vi "SetWindowFullscreen.vi"(8 "No Error":errorcluster, 10 "Fullscreen":bool, 11 "Window [SDL_Window *]":i64 format="%.0x") -> (0 "Error Out":errorcluster)   [LabVIEW 2026, in "SDL3.lvlib" / "Video.lvlib"]
doc: "<B>Summary</B>\nRequest that the window's fullscreen state be changed.\n\n<B>Remarks</B>\nBy default a window in fullscreen state uses borderless fullscreen desktop mode, but a specific exclusive display mode can be set using <B>SDL_SetWindowFullscreenMode()</B>.\n\nOn some windowing systems this request is asynchronous and the new fullscreen state may not have have been applied immediately upon the return of this function. If an immediate change is required, call <B>SDL_SyncWindow()</B> to block until the changes have taken effect.\n\nWhen the window state changes, an <B>SDL_EVENT_WINDOW_ENTER_FULLSCREEN</B> or <B>SDL_EVENT_WINDOW_LEAVE_FULLSCREEN</B> event will be emitted. Note that, as this is just a request, it can be denied by the windowing system."
uses:
  Video.lvlib
  <vilib>/Utility/error.llb/Error Cluster From Error Code.vi
  Error/Error.lvlib
  Lib/SDL3.dll
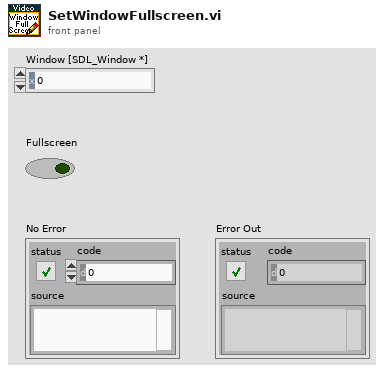
[diagram p1: front panel]
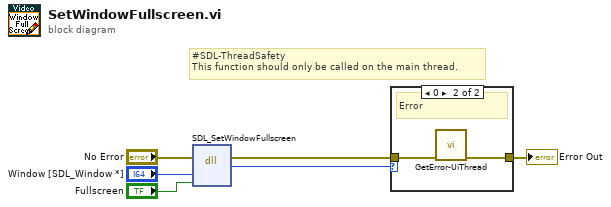
[diagram p0: block diagram]
diagram:
  # "#SDL-ThreadSafety\nThis function should only be called on the main thread."
  n1 = dll-call lib="C:/Users/saukko/Dev/LV-SDL3/Sources/SDL3/Lib/SDL3.*" fn="SDL_SetWindowFullscreen"(error in="No Error", "window"="Window [SDL_Window *]", "on_top"="Fullscreen") -> (error out=w3:errorcluster, "return type"=w2:i32)  [unwired: 4 in, 1 out]
  n2 = case shown="0" w2 {
    tunnel: w3 -> [w7 w9]
    tunnel: [w7 w8] -> w5
    frame Default {
      # "Ok"
    }
    frame 0 {
      # "Error"
      n3 = call "GetError-UiThread.vi"("No Error"=w9) -> ("error out"=w8:errorcluster)  [unwired: 10 in]
    }
  }
  "Error Out" <- w5
